vi "Roller Mode Select.vi"() -> (3 "Mode":T1)   [LabVIEW 2015]
uses:
  Common Code/Roller Mode Enum.ctl
  Robot Global Data.vi
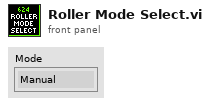
[diagram p1: front panel]
types:
  T1 = typedef "Roller Mode Enum.ctl" = enum16{"Manual", "Safe", "Auto"}
  T2 = enum16{"0", "1", "2", "3", "4", "5", "6", "7", "8", "9", "A", "B", "C", "D", "E", "F", "G", "H", "I", "J", "K", "L", "M", "N", "O", "P", "Q", "R", "S", "T", "U", "V", "W", "X", "Y", "Z", "F1", "F2", "F3", "F4", "F5", "F6", "F7", "F8", "F9", "F10", "F11", "F12", "F13", "F14", "F15", "ADD", "BACK", "BACKSLASH", "CAPITAL", "COMMA", "DECIMAL", "DELETE", "DIVIDE", "DOWN", "END", "EQUALS", "ESCAPE", "GRAVE (`)", "HOME", "INSERT", "LBRACKET", "LCONTROL", "LEFT", "L ALT", "LSHIFT", "LWIN", "MINUS", "MULTIPLY", "NEXT", "NUMLOCK", "NUMPAD_0", "NUMPAD_1", "NUMPAD_2", "NUMPAD_3", "NUMPAD_4", "NUMPAD_5", "NUMPAD_6", "NUMPAD_7", "NUMPAD_8", "NUMPAD_9", "PAUSE", "PERIOD", "PRIOR (PG UP)", "RBRACKET", "RCONTROL", "RETURN", "RIGHT", "R ALT", "RSHIFT", "RWIN", "SCROLL", "SEMICOLON", "SLASH", "SPACE", "SUBTRACT", "TAB", "UP", "ENTER (num pad)", "' (quote)"}
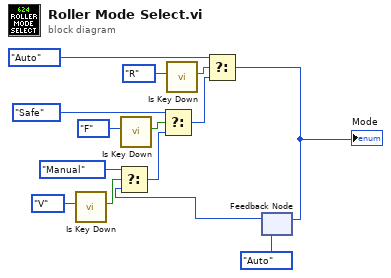
[diagram p0: block diagram]
diagram:
  n1 = call "Is Key Down.vi"("Key"=T2."V") -> ("Key Down?"=w9:bool)  [unwired: 10 in]
  n2 = call "Is Key Down.vi"("Key"=T2."F") -> ("Key Down?"=w8:bool)  [unwired: 10 in]
  n3 = call "Is Key Down.vi"("Key"=T2."R") -> ("Key Down?"=w7:bool)  [unwired: 10 in]
  n4 = feedback #1(Roller_Mode_Enum."Auto" ("Mode")) -> (w2:T1)
  n5 = Select(t=Roller_Mode_Enum."Manual" ("Mode"), s=w9, f=w2) -> (s? t:f=w14:T1)
  n6 = Select(t=Roller_Mode_Enum."Safe" ("Mode"), s=w8, f=w14) -> (s? t:f=w13:T1)
  n7 = Select(t=Roller_Mode_Enum."Auto" ("Mode"), s=w7, f=w13) -> (s? t:f=w1:T1)
  "Mode" <- w1
  n8 = feedback-in #1(w1) -> ()
